vi "Configure Marker Characteristics.vi"(6 "Band Right Edge Frequency (0 Hz)":dbl, 7 "Band Left Edge Frequency (0 Hz)":dbl, 8 "error in (no error)":errorcluster, 9 "Marker Function (0: Off)":i32(ring) items=["Off", "Marker Noise", "Band Power", "Band Density"], 10 "Active Marker (1: Marker1)":i32(ring)=1 items=["Marker1"=1, "Marker2"=2, "Marker3"=3, "Marker4"=4, "Marker5"=5, "Marker6"=6, "Marker7"=7, "Marker8"=8, "Marker9"=9, "Marker10"=10, "Marker11"=11, "Marker12"=12], 11 "VISA resource name":refnum<visa-resource-name>) -> (0 "error out":errorcluster, 3 "VISA resource name out":refnum<visa-resource-name>)   [LabVIEW 2018, in "Agilent MXA Series.lvlib"]
doc: "Configures the marker settings on the spectrum analyzer, such as Marker Function.\n\n<B>Note:</B>\nYou can use this VI only under Swept SA measurement type."
uses:
  Agilent MXA Series.lvlib
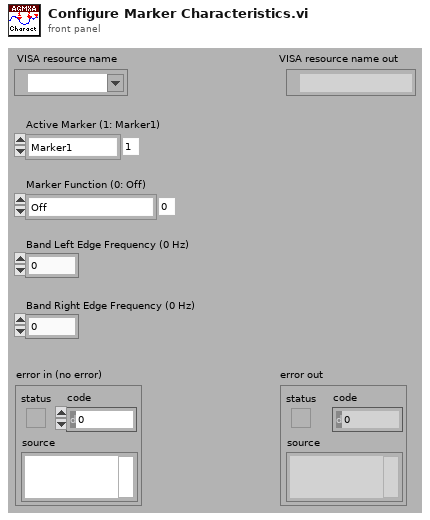
[diagram p1: front panel]
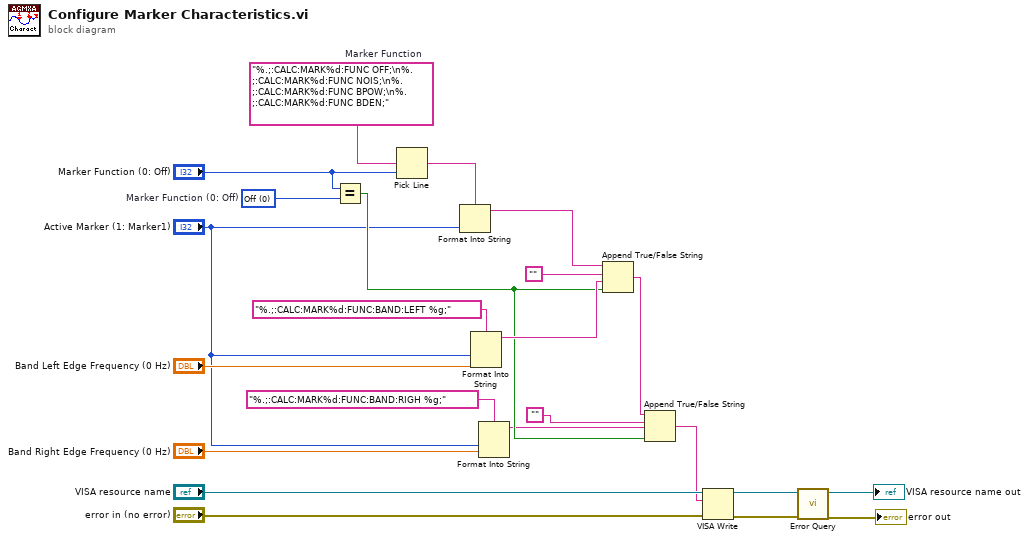
[diagram p0: block diagram]
diagram:
  w1 = 0 items=["Off", "Marker Noise", "Band Power", "Band Density"]  # Marker Function (0: Off)
  w23 = "%.;:CALC:MARK%d:FUNC OFF;\n%.;:CALC:MARK%d:FUNC NOIS;\n%.;:CALC:MARK%d:FUNC BPOW;\n%.;:CALC:MARK%d:FUNC BDEN;"  # Marker Function
  n1 = Equal?(x="Marker Function (0: Off)", y=w1) -> (x = y?=w16:bool)
  n2 = Pick Line(multi-line string=w23, line index="Marker Function (0: Off)") -> (output string=w22:string)  [unwired: 1 in]
  n3 = Format Into String(format string=w22, "Active Marker (1: Marker1)") -> (resulting string=w20:string)  [unwired: 2 in, 1 out]
  n4 = Format Into String(format string="%.;:CALC:MARK%d:FUNC:BAND:LEFT %g;", "Active Marker (1: Marker1)", "Band Left Edge Frequency (0 Hz)") -> (resulting string=w19:string)  [unwired: 2 in, 1 out]
  n5 = Format Into String(format string="%.;:CALC:MARK%d:FUNC:BAND:RIGH %g;", "Active Marker (1: Marker1)", "Band Right Edge Frequency (0 Hz)") -> (resulting string=w15:string)  [unwired: 2 in, 1 out]
  n6 = Append True/False String(1:w16, 2:w19, 3:"" ("true string"), 4:w20) -> (0:w13:string)
  n7 = Append True/False String(1:w16, 2:w15, 3:"" ("true string"), 4:w13) -> (0:w6:string)
  n8 = VISA Write(VISA resource name="VISA resource name", write buffer=w6, error in (no error)="error in (no error)") -> (VISA resource name out=w12:refnum<visa-resource-name>, error out=w11:errorcluster)  [unwired: 1 out]
  n9 = call "Error Query.vi"("error in (no error)"=w11, "VISA resource name"=w12) -> ("error out"=→"error out":errorcluster, "VISA resource name out"=→"VISA resource name out":refnum<visa-resource-name>)  [unwired: 6 in, 2 out]
